vi "Rohde & Schwarz VNA Find Memory Trace.vi"(6 "Channel":i8=1 min=1 max=99 step=1, 7 "Rohde & Schwarz VNA":T1, 8 "error in (no error)":errorcluster, 11 "VISA Resource Name":refnum<visa-resource-name>) -> (0 "error out":errorcluster, 2 "Memory Exists?":bool, 3 "dup VISA Resource Name":refnum<visa-resource-name>)   [LabVIEW 2011]
doc: "It is recommended that you hold off triggers before running this VI as the HP8753 tends to \"hang\" if data is read while measurements are being taken.\n\n This VI is used to collect and display data generated by the HP8753 Network Analyzer. The VI can display error-corrected data, error-corrected trace memory, fully formatted data and memory traces. For further information on these types of data see Processsing Chain figure in the HPIB programming note. When the data type is a formatted data, the instruments screen will change to reflect what is being displayed, eg. selecting \"formatted memory\" changes the display to \"MEMORY\".\n\n The data values shown depend upon the data type and the measurement format. If the data type is \"error-corrected data\" or \"error-corrected trace memory\" and/or the measurement format is \"Smith chart\" or \"polar\", the data values are real,imaginary pairs. Otherwise the data values are stimulus,response pairs. These pairs correspond to what is shown in the graphical display.\n\n Data can also be saved to a file with this VI. When saving a file, the stimulus is always shown. The real,imaginary components or the response value are also shown depending upon the data type and the measurement format. \n\n No units are shown on the VI front panel or in the data file. All units are basic units of Hz, dB, seconds, ohms, etc. The \"saved data comments\" control should be used for any special information such as the measurement format, averaging and smoothing information, etc.\n\n Whether or not data is saved and whether the output is in real,imaginary pairs or stimulus,response parirs affects the speed of this VI. When data is saved to a file and/or when data is in stimulus,response pairs, requires the reading of the stimulus values which slows the VI down. The fastest reads are done when the data type is \"error-corrected data\" or \"error-corrected trace memory\" and/or the measurement format is \"Smith chart\" or \"polar\" and data is not being saved to a file.\n\n This VI sets the format, ie. linear or logarithmic, depending upon the sweep type. \n\nFYI - Originally this VI was written without considering the stimulus values. In most case this would be fine for display purposes as the point number could be used for the X value as most sweeps are evenly spaced. This is not the case with frequency list sweeps which can have big gaps in the sweep. For this reason the stimulus value is read (at least in the cases explained above) to make the LabVIEW display match what is display on the instrument's display."
uses:
  TypeDefs/Rohde & Schwarz VNA Instrument Info.ctl
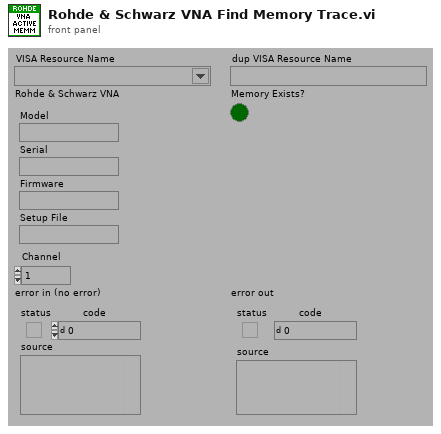
[diagram p1: front panel]
types:
  T1 = typedef "Rohde & Schwarz VNA Instrument Info.ctl" = cluster{"Model":string, "Serial":string, "Firmware":string, "Setup File":string}
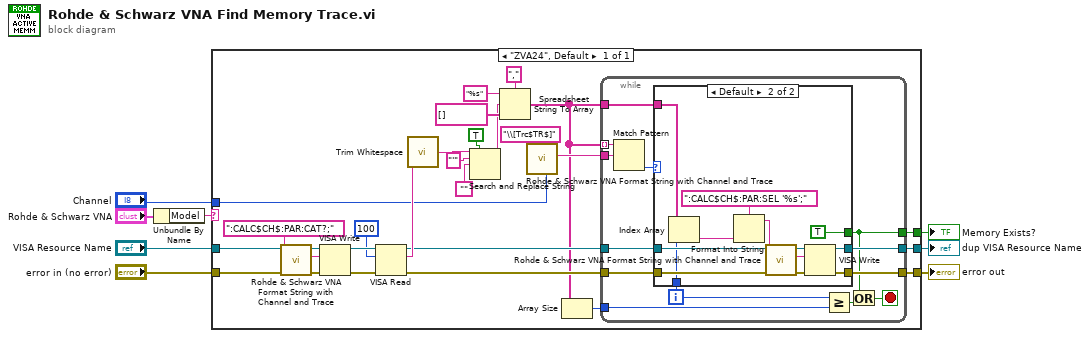
[diagram p0: block diagram]
diagram:
  n1 = Unbundle By Name("Rohde & Schwarz VNA") -> ("Model"=w2:string)
  n2 = case shown="\"ZVA24\", Default" w2 {
    tunnel: "VISA Resource Name" -> [w34]
    tunnel: "Channel" -> [w18]
    tunnel: "error in (no error)" -> [w17]
    tunnel: [w13] -> w5
    tunnel: [w14] -> w4
    tunnel: [w12] -> w1
    frame "ZVA24", Default {
      n3 = call "Rohde & Schwarz VNA Format String with Channel and Trace.vi"("String"=":CALC$CH$:PAR:CAT?;" ("write buffer")) -> ("String Out"=w31:string)  [unwired: 2 in, 6 out]
      n4 = VISA Write(VISA resource name=w34, write buffer=w31, error in (no error)=w17) -> (VISA resource name out=w33:refnum<visa-resource-name>, error out=w21:errorcluster)  [unwired: 1 out]
      n5 = VISA Read(VISA resource name=w33, byte count=u32 100, error in (no error)=w21) -> (VISA resource name out=w16:refnum<visa-resource-name>, read buffer=w22:string, error out=w15:errorcluster)  [unwired: 1 out]
      n6 = call <vilib>:"Trim Whitespace.vi"("string"=w22) -> ("trimmed string"=w23:string)  [unwired: 1 in]
      n7 = Search and Replace String(replace all?=TRUE ("replace all? (F)"), input string=w23, search string="'", replace string="") -> (result string=w24:string)  [unwired: 1 in, 6 out]
      n8 = Spreadsheet String To Array(delimiter (Tab)=",", format string="%s", spreadsheet string=w24, array type (2D Dbl)=string[] []) -> (array=w9:string[])
      n9 = call "Rohde & Schwarz VNA Format String with Channel and Trace.vi"("Trace"=w18, "String"="\\[Trc$TR$]") -> ("String Out"=w11:string)  [unwired: 1 in, 6 out]
      n10 = Array Size(array=w9) -> (size(s)=w10:i32)
      n11 = while {
        tunnel: w9 -> [w43] mode=indexing
        tunnel: w16 -> [w47]
        tunnel: w15 -> [w46]
        tunnel: [w45] -> w14
        tunnel: [w44] -> w13
        tunnel: [w40] -> w12
        tunnel: w11 -> [w42]
        tunnel: w10 -> [w38]
        tunnel: w9 -> [w36]
        i -> [w35]
        stop <- w39 stop-if-true
        n12 = Match Pattern(string=w43, regular expression=w42) -> (offset past match=w41:i32)  [unwired: 4 out]
        n13 = case shown="Default" w41 {
          tunnel: w36 -> [_ w59]
          tunnel: w47 -> [w49 w60]
          tunnel: w46 -> [w48 w57]
          tunnel: [w49 w51] -> w45
          tunnel: [w48 w50] -> w44
          tunnel: [_ TRUE ("Memory Exists?")] -> w40
          tunnel: w35 -> [_ w52]
          frame -1 {
          }
          frame Default {
            n14 = Index Array(array=w59, index=w52) -> (element=w56:string)
            n15 = Format Into String(format string=":CALC$CH$:PAR:SEL '%s';" ("write buffer"), w56) -> (resulting string=w54:string)  [unwired: 2 in, 1 out]
            n16 = call "Rohde & Schwarz VNA Format String with Channel and Trace.vi"("String"=w54) -> ("String Out"=w58:string)  [unwired: 2 in, 6 out]
            n17 = VISA Write(VISA resource name=w60, write buffer=w58, error in (no error)=w57) -> (VISA resource name out=w51:refnum<visa-resource-name>, error out=w50:errorcluster)  [unwired: 1 out]
          }
        }
        n18 = Greater Or Equal?(x=w35, y=w38) -> (x >= y?=w37:bool)
        n19 = Or(x=w40, y=w37) -> (x .or. y?=w39:bool)
      }
    }
  }
  "dup VISA Resource Name" <- w4
  "error out" <- w5
  "Memory Exists?" <- w1
